vi "get selftest.vi"(8 "error in (no error)":errorcluster, 11 "VISA resource name":refnum<visa-resource-name>) -> (0 "error out":errorcluster, 1 "accel selftest":dbl[](array[numeric]), 2 "gyro selftest":dbl[](array[numeric]), 3 "VISA resource out":refnum<visa-resource-name>)   [LabVIEW 2013]
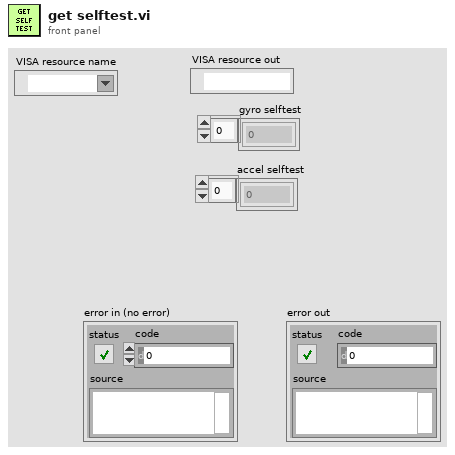
[diagram p1: front panel]
types:
  T1 = typedef "selftest_data.ctl" = cluster{"gyro_trim":u8[], "gyro_selftest":i16[], "gyro_base":i16[], "accel_trim":u8[], "accel_selftest":i16[], "accel_base":i16[]}
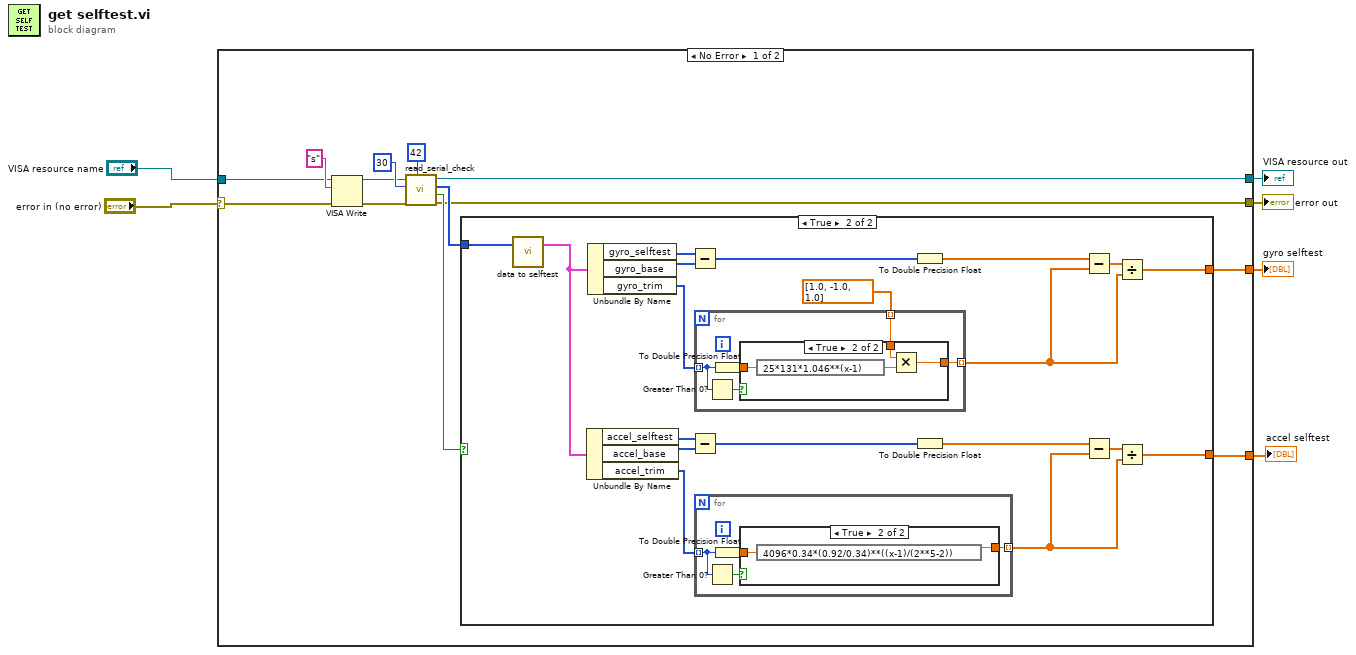
[diagram p0: block diagram]
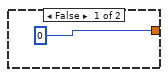
[diagram p3: hidden frame]
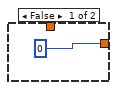
[diagram p4: hidden frame]
diagram:
  n1 = case shown="No Error" "error in (no error)" {
    selector: "error in (no error)" -> [w14 w56]
    tunnel: "VISA resource name" -> [w13 w57]
    tunnel: [w10 _] -> w4
    tunnel: [w9 _] -> w3
    tunnel: [w8 w57] -> w1
    tunnel: [w7 w56] -> w2
    frame No Error {
      n2 = VISA Write(VISA resource name=w13, write buffer="s", error in (no error)=w14) -> (VISA resource name out=w17:refnum<visa-resource-name>, error out=w15:errorcluster)  [unwired: 1 out]
      n3 = call "read_serial_check.vi"("checkval"=u8 42, "error in (no error)"=w15, "byte count"=u32 30, "VISA resource name"=w17) -> ("error out"=w7:errorcluster, "good"=w11:bool, "data"=w12:u8[], "VISA resource out"=w8:refnum<visa-resource-name>)  [unwired: 4 in]
      n4 = case shown="True" w11 {
        tunnel: w12 -> [_ w36]
        tunnel: [_ w29] -> w10
        tunnel: [_ w20] -> w9
        frame False {
        }
        frame True {
          n5 = call "data to selftest.vi"("byte array"=w36) -> ("selftest"=w21:T1)  [unwired: 2 in]
          n6 = Unbundle By Name(w21) -> ("accel_selftest"=w22:i16[], "accel_base"=w23:i16[], "accel_trim"=w24:u8[])
          n7 = Unbundle By Name(w21) -> ("gyro_selftest"=w38:i16[], "gyro_base"=w37:i16[], "gyro_trim"=w34:u8[])
          n8 = Subtract(x=w38, y=w37) -> (x-y=w33:i16[])
          n9 = Subtract(x=w22, y=w23) -> (x-y=w25:i16[])
          n10 = for {
            tunnel: w34 -> [w49] mode=indexing
            tunnel: [w48] -> w30 mode=indexing
            tunnel: dbl[] [1.0, -1.0, 1.0] ("gyro_trim") -> [w46] mode=indexing
            n11 = Greater Than 0?(x=w49) -> (x > 0?=w50:bool)
            n12 = To Double Precision Float(number=w49) -> (double precision float=w47:dbl)
            n13 = case shown="True" w50 {
              tunnel: w47 -> [_ w55]
              tunnel: [0 w54] -> w48
              tunnel: w46 -> [_ w52]
              frame False {
              }
              frame True {
                n14 = expression code="25*131*1.046**(x-1)"(w55) -> (w53:dbl)
                n15 = Multiply(x=w52, y=w53) -> (x*y=w54:dbl)
              }
            }
          }
          n16 = for {
            tunnel: w24 -> [w41] mode=indexing
            tunnel: [w40] -> w28 mode=indexing
            n17 = Greater Than 0?(x=w41) -> (x > 0?=w42:bool)
            n18 = To Double Precision Float(number=w41) -> (double precision float=w39:dbl)
            n19 = case shown="True" w42 {
              tunnel: w39 -> [_ w45]
              tunnel: [0 w44] -> w40
              frame False {
              }
              frame True {
                n20 = expression code="4096*0.34*(0.92/0.34)**((x-1)/(2**5-2))"(w45) -> (w44:dbl)
              }
            }
          }
          n21 = To Double Precision Float(number=w33) -> (double precision float=w32:dbl[])
          n22 = To Double Precision Float(number=w25) -> (double precision float=w26:dbl[])
          n23 = Subtract(x=w32, y=w30) -> (x-y=w31:dbl[])
          n24 = Subtract(x=w26, y=w28) -> (x-y=w27:dbl[])
          n25 = Divide(x=w31, y=w30) -> (x/y=w29:dbl[])
          n26 = Divide(x=w27, y=w28) -> (x/y=w20:dbl[])
        }
      }
    }
    frame Error {
    }
  }
  "gyro selftest" <- w4
  "accel selftest" <- w3
  "error out" <- w2
  "VISA resource out" <- w1
